vi "Read data_tool offset data.vi"(11 "path":path) -> (3 "offset":T1)   [LabVIEW 2016]
uses:
  <vilib>/Utility/file.llb/Read Delimited Spreadsheet (string).vi
  <vilib>/Utility/file.llb/Read Delimited Spreadsheet (DBL).vi
panel:
  out "Tool Offsets":T2
  out "subarray":string[](array[string])
  out "path 2":path
  out "Tool Offset datas":T3
  out "error out":errorcluster
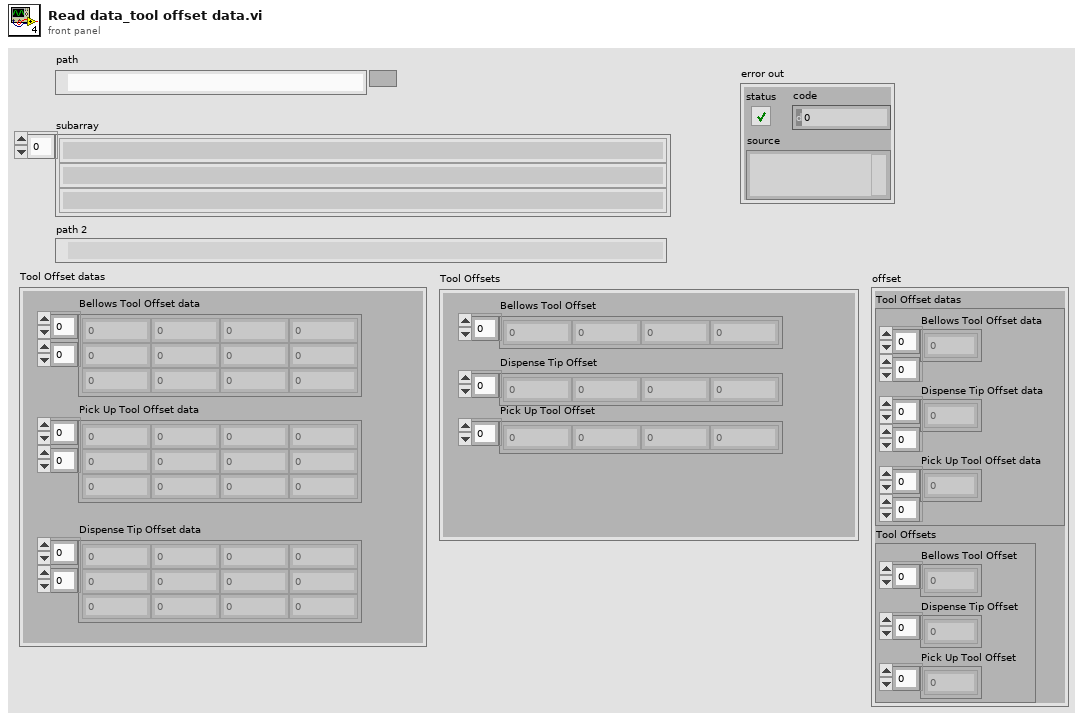
[diagram p1: front panel]
types:
  T1 = cluster{"Tool Offset datas":cluster{"Bellows Tool Offset data":dbl[][], "Dispense Tip Offset data":dbl[][], "Pick Up Tool Offset data":dbl[][]}, "Tool Offsets":cluster{"Bellows Tool Offset":dbl[], "Dispense Tip Offset":dbl[], "Pick Up Tool Offset":dbl[]}}
  T2 = cluster{"Bellows Tool Offset":dbl[], "Dispense Tip Offset":dbl[], "Pick Up Tool Offset":dbl[]}
  T3 = cluster{"Bellows Tool Offset data":dbl[][], "Dispense Tip Offset data":dbl[][], "Pick Up Tool Offset data":dbl[][]}
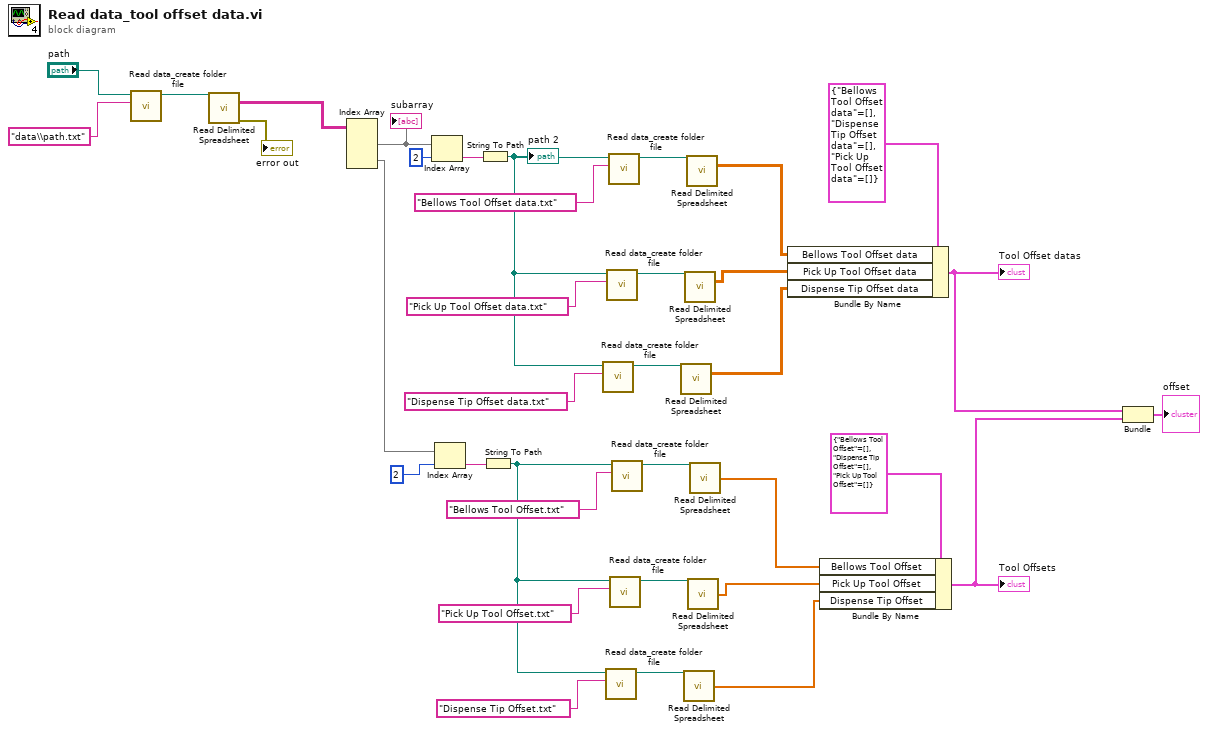
[diagram p0: block diagram]
diagram:
  n1 = call "Read data_create folder file.vi"("name or relative path"="data\\path.txt", "path"="path") -> ("dup path"=w35:path)  [unwired: 9 in]
  n2 = call-poly <vilib>:"Read Delimited Spreadsheet.vi"("file path (dialog if empty)"=w35) -> ("all rows"=w34:string[][], "error out"=→"error out":errorcluster)  [unwired: 9 in, 4 out]
  n3 = Index Array(array=w34) -> (element #1=w31:string[], element #2=w8:string[])  [unwired: 4 in]
  "subarray" <- w31
  n4 = Index Array(array=w31, index=2) -> (element=w30:string)
  n5 = Index Array(array=w8, index=2) -> (element=w9:string)
  n6 = String To Path(string=w30) -> (path=w18:path)
  "path 2" <- w18
  n7 = String To Path(string=w9) -> (path=w17:path)
  n8 = call "Read data_create folder file.vi"("name or relative path"="Dispense Tip Offset data.txt", "path"=w18) -> ("dup path"=w27:path)  [unwired: 9 in]
  n9 = call "Read data_create folder file.vi"("name or relative path"="Dispense Tip Offset.txt", "path"=w17) -> ("dup path"=w12:path)  [unwired: 9 in]
  n10 = call "Read data_create folder file.vi"("name or relative path"="Pick Up Tool Offset data.txt", "path"=w18) -> ("dup path"=w28:path)  [unwired: 9 in]
  n11 = call "Read data_create folder file.vi"("name or relative path"="Bellows Tool Offset data.txt", "path"=w18) -> ("dup path"=w29:path)  [unwired: 9 in]
  n12 = call "Read data_create folder file.vi"("name or relative path"="Pick Up Tool Offset.txt", "path"=w17) -> ("dup path"=w11:path)  [unwired: 9 in]
  n13 = call "Read data_create folder file.vi"("name or relative path"="Bellows Tool Offset.txt", "path"=w17) -> ("dup path"=w10:path)  [unwired: 9 in]
  n14 = call-poly <vilib>:"Read Delimited Spreadsheet.vi"("file path (dialog if empty)"=w27) -> ("all rows"=w23:dbl[][])  [unwired: 9 in, 5 out]
  n15 = call-poly <vilib>:"Read Delimited Spreadsheet.vi"("file path (dialog if empty)"=w12) -> ("first row"=w4:dbl[])  [unwired: 9 in, 5 out]
  n16 = call-poly <vilib>:"Read Delimited Spreadsheet.vi"("file path (dialog if empty)"=w28) -> ("all rows"=w24:dbl[][])  [unwired: 9 in, 5 out]
  n17 = call-poly <vilib>:"Read Delimited Spreadsheet.vi"("file path (dialog if empty)"=w29) -> ("all rows"=w25:dbl[][])  [unwired: 9 in, 5 out]
  n18 = call-poly <vilib>:"Read Delimited Spreadsheet.vi"("file path (dialog if empty)"=w11) -> ("first row"=w5:dbl[])  [unwired: 9 in, 5 out]
  n19 = call-poly <vilib>:"Read Delimited Spreadsheet.vi"("file path (dialog if empty)"=w10) -> ("first row"=w6:dbl[])  [unwired: 9 in, 5 out]
  n20 = Bundle By Name(cluster=T3 {"Bellows Tool Offset data"=[], "Dispense Tip Offset data"=[], "Pick Up Tool Offset data"=[]} ("Tool Offset datas"), "Bellows Tool Offset data"=w25, "Pick Up Tool Offset data"=w24, "Dispense Tip Offset data"=w23) -> (w3:T3)
  "Tool Offset datas" <- w3
  n21 = Bundle By Name(cluster=T2 {"Bellows Tool Offset"=[], "Dispense Tip Offset"=[], "Pick Up Tool Offset"=[]} ("Tool Offsets"), "Bellows Tool Offset"=w6, "Pick Up Tool Offset"=w5, "Dispense Tip Offset"=w4) -> (w2:T2)
  "Tool Offsets" <- w2
  n22 = Bundle("Tool Offset datas"=w3, "Tool Offsets"=w2) -> (→"offset":T1)  [unwired: 1 in]
